vi "FTW-TransferClient-S3-ProcessUpload.vi"(8 "Upload Request":refnum<k24>, 9 "Transfer Status":refnum<user-event>, 10 "Initial Time":u32, 11 "Transfer Utility":refnum<k24>) -> ()   [LabVIEW 2013, in "FTW-TransferClient-S3.lvclass"]
uses:
  FTW-TransferClient-S3.lvclass
  C:/Jobs/Tools/featherweight-trunk/Windows/src/Transfer Client/S3/AWSSDK.dll
  AWSSDK.dll
  FTW-TransferClient-TransferStatus.ctl
  FTW-TransferClient.lvclass
panel:
  # "Inputs"
  # "Outputs"
  # "No Outputs - this VI\nis fire and forget"
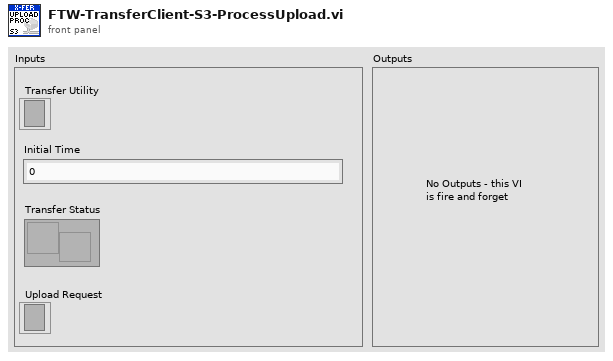
[diagram p1: front panel]
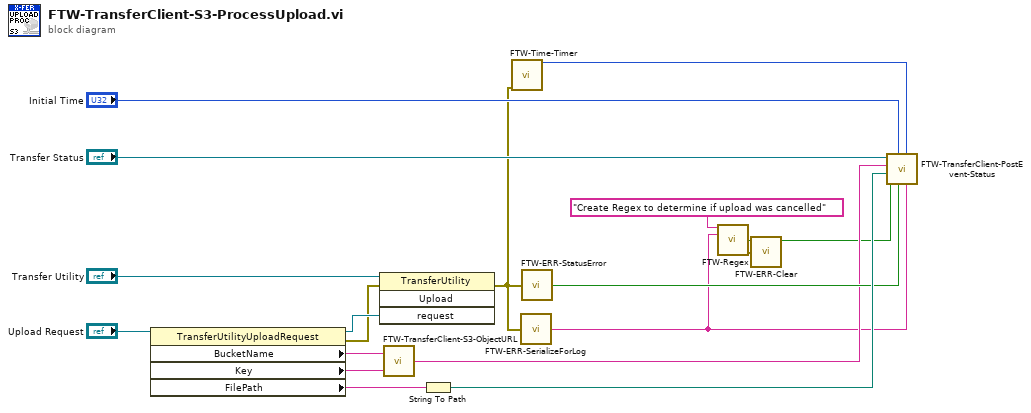
[diagram p0: block diagram]
diagram:
  n1 = property class="TransferUtilityUploadRequest"(reference="Upload Request") -> (reference out=w11:refnum<k24>, error out=w10:errorcluster, "BucketName"=w9:string, "Key"=w8:string, "FilePath"=w18:string)  [unwired: 1 in]
  n2 = invoke class="TransferUtility" method="Upload"(reference="Transfer Utility", error in=w10, "request"=w11) -> (error out=w2:errorcluster)  [unwired: 1 in, 3 out]
  n3 = call "FTW-TransferClient-S3-ObjectURL.vi"("Object Bucket"=w9, "Object Key"=w8) -> ("Object URL"=w7:string)  [unwired: 2 in]
  n4 = String To Path(string=w18) -> (path=w14:path)
  n5 = call "FTW-Time-Timer.vi"("error in"=w2) -> ("Current Tick Count"=w12:u32)  [unwired: 12 in, 2 out]
  n6 = call "FTW-ERR-SerializeForLog.vi"("error in"=w2) -> ("Serialized Error"=w1:string)
  n7 = call "FTW-ERR-StatusError.vi"("error to check"=w2) -> ("Error?"=w13:bool)
  n8 = call "FTW-Regex.vi"("Regular Expression"="Create Regex to determine if upload was cancelled", "Input String"=w1) -> ("Match Found?"=w4:bool, "error out"=w3:errorcluster)  [unwired: 9 in, 3 out]
  n9 = call "FTW-ERR-Clear.vi"("error to snuff"=w3) -> ()  [unwired: 1 out]
  n10 = call "FTW-TransferClient-PostEvent-Status.vi"("Error Message"=w1, "Timestamp"=w12, "Error?"=w13, "Initial Timestamp"="Initial Time", "Cancelled?"=w4, "Local Filepath"=w14, "Remote URI"=w7, "Transfer Status Event"="Transfer Status") -> ()  [unwired: 4 in]
